vi "CAN_Heartbeat_switch.vi"(8 "error in":errorcluster, 11 "Enable? (T)":bool=TRUE) -> (0 "error out":errorcluster)   [LabVIEW 2009, in "OWNCAN.lvlib"]
doc: "Swithes heartbeat signal (on/off)"
uses:
  OWNCAN.lvlib
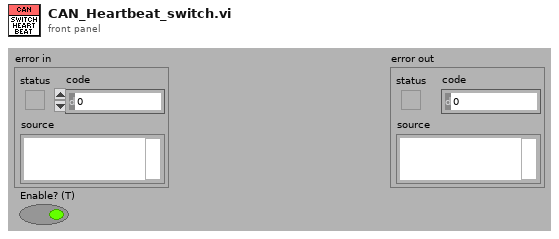
[diagram p1: front panel]
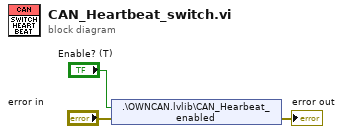
[diagram p0: block diagram]
diagram:
  n1 = shared-variable ".\\OWNCAN.lvlib\\CAN_Hearbeat_enabled"("Enable? (T)", error in="error in") -> (error out=→"error out":errorcluster)
